vi "Read Device Type.vi"(8 "error in (no error)":errorcluster, 11 "heater_flow_synthesiser in":refnum<class "heater_flow_synthesiser.lvclass">) -> (0 "error out":errorcluster, 2 "Device Type":string, 3 "heater_flow_synthesiser out":refnum<class "heater_flow_synthesiser.lvclass">)   [LabVIEW 2020, in "polar_bear_plus_drivers.lvlib" / "heater_flow_synthesiser.lvclass"]
doc: "Get the device type string used to identify this driver class."
uses:
  <instrlib>/RxnRover/Driver Polar Bear Plus/heater_flow_synthesiser/heater_flow_synthesiser.lvclass
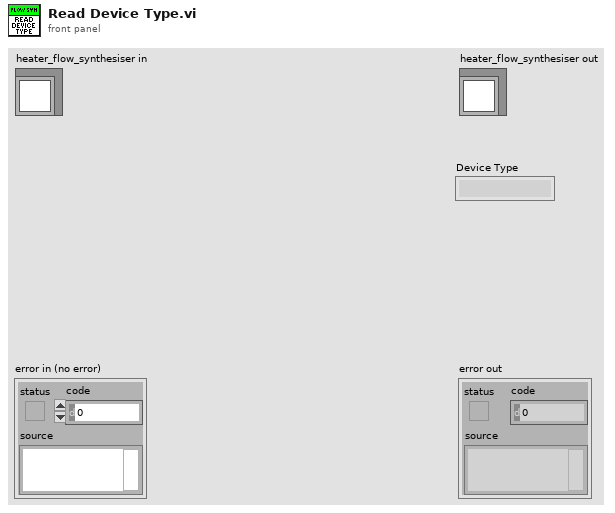
[diagram p1: front panel]
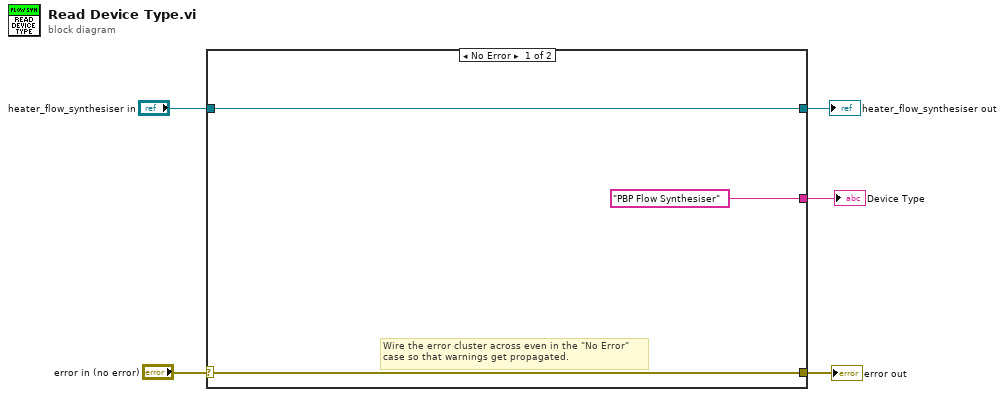
[diagram p0: block diagram]
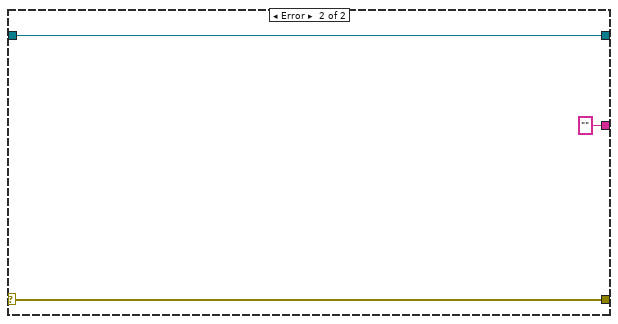
[diagram p2: hidden frame]
diagram:
  n1 = case shown="No Error" "error in (no error)" {
    selector: "error in (no error)" -> [w7 w11]
    tunnel: [w7 w11] -> w5
    tunnel: [w8 w10] -> w3
    tunnel: "heater_flow_synthesiser in" -> [w8 w10]
    tunnel: ["PBP Flow Synthesiser" ""] -> w4
    frame No Error {
      # "Wire the error cluster across even in the \"No Error\"\ncase so that warnings get propagated."
    }
    frame Error {
    }
  }
  "error out" <- w5
  "heater_flow_synthesiser out" <- w3
  "Device Type" <- w4
